vi "FGV_UsersDatabase.vi"(7 "Database action (read data)":T2=enum."Read data", 8 "error in (no error)":errorcluster, 11 "User":T1) -> (0 "error out":errorcluster, 3 "Users Data":T1[](array[typedef]))   [LabVIEW 2020]
uses:
  #typedef_User.ctl
  #typedef_FGV_DatabaseAction.ctl
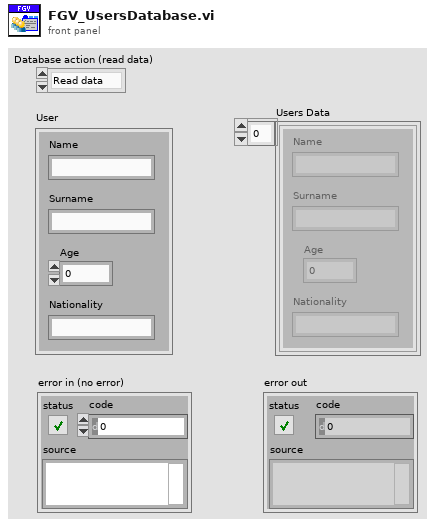
[diagram p1: front panel]
types:
  T1 = typedef "#typedef_User.ctl" = cluster{"Name":string, "Surname":string, "Age":dbl, "Nationality":string}
  T2 = typedef "#typedef_FGV_DatabaseAction.ctl" = enum16{"Add user", "Read data", "Clear data"}
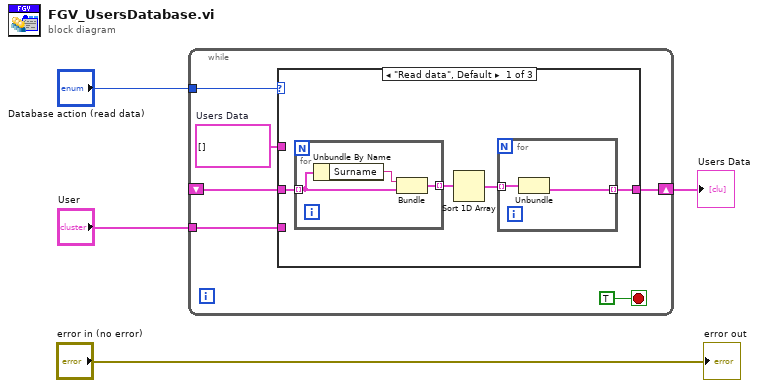
[diagram p0: block diagram]
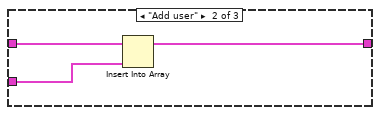
[diagram p2: hidden frame]
diagram:
  n1 = while {
    tunnel: "Database action (read data)" -> [w9]
    shift-right: [w7] -> w3
    shift-left: _ -> [w6]
    tunnel: "User" -> [w5]
    stop <- TRUE stop-if-true
    w8 = T1[] []  # Users Data
    n2 = case shown="\"Read data\", Default" w9 {
      tunnel: w8 -> [_ _ w23]
      tunnel: [w11 w20 w23] -> w7
      tunnel: w6 -> [w14 w22 _]
      tunnel: w5 -> [_ w21 _]
      frame "Read data", Default {
        n3 = for {
          tunnel: w14 -> [w18] mode=indexing
          tunnel: [w17] -> w13 mode=indexing
          n4 = Unbundle By Name(w18) -> ("Surname"=w19:string)
          n5 = Bundle("Surname"=w19, "Cluster 2"=w18) -> (w17:cluster{"Surname":string, "Cluster 2":T1})  [unwired: 1 in]
        }
        n6 = Sort 1D Array(array=w13) -> (sorted array=w12:cluster{"Surname":string, "Cluster 2":T1}[])
        n7 = for {
          tunnel: w12 -> [w16] mode=indexing
          tunnel: [w15] -> w11 mode=indexing
          n8 = Unbundle(w16) -> ("Cluster 2"=w15:T1)  [unwired: 1 out]
        }
      }
      frame "Add user" {
        n9 = Insert Into Array(array=w22, new element=w21) -> (w20:T1[])  [unwired: 1 in]
      }
      frame "Clear data" {
      }
    }
  }
  "Users Data" <- w3
  "error out" <- "error in (no error)"
